vi "ClickConfocalSpot.vi"() -> ()   [LabVIEW 2013]
uses:
  <vilib>/Platform/TimedLoop/XDataNode/wakeup.ctl
  <vilib>/Platform/TimedLoop/XDataNode/XDNodeRunTimeDep.lvlib
  <vilib>/Platform/TimedLoop/XDataNode/nitl_modes.ctl
  <vilib>/Platform/TimedLoop/XDataNode/timing_clust.ctl
  <vilib>/Platform/TimedLoop/XDataNode/XDataNode.xnode
  <vilib>/Utility/miscctls.llb/LVPoint32TypeDef.ctl
  <vilib>/Utility/miscctls.llb/LVMinMaxIncTypeDef.ctl
panel:
  in  "BD 2 Frequency 2 (MHz)":dbl=26.0 min=60.0 max=90.0 step=1.0 format="%#_6p"
  in  "BD 1 Frequency 2 (MHz)":dbl=90.0 caption="T2 X (MHz)" min=60.0 max=90.0 step=1.0 format="%#_6p"
  in  "BD 2 Frequency 3 (MHz)":dbl=26.0 min=60.0 max=90.0 step=1.0 format="%#_6p"
  in  "BD 1 Frequency 3 (MHz)":dbl=70.0 min=60.0 max=90.0 step=1.0 format="%#_6p"
  in  "Trap Delta (MHz)":dbl=20.0 step=1.0
  out "X RF Frequency Limits (MHz)":T1={"Minimum"=60.0, "Maximum"=90.0, "Increment"=1.0}
  out "Y RF Frequency Limits (MHz)":T1={"Minimum"=60.0, "Maximum"=90.0, "Increment"=1.0}
  out "Manipulating Trap":bool
  in  "BD 1 Frequency 1 (MHz)":dbl=70.0 caption="T1 X (MHz)" min=60.0 max=90.0 step=1.0 format="%#_6p"
  in  "BD 2 Frequency 1 (MHz)":dbl=26.0 min=60.0 max=90.0 step=1.0 format="%#_6p"
  out "Initial Y":dbl=2.5691326639606933
  out "Initial X":dbl=1.6310662274449115
  in  "Scan steps (MCL)":u64=40 caption="Scan steps (x)"
  in  "Scan lines (y)":u64=20
  out "Actual MCL Inc (V)":dbl=0.14099551377910702
  out "Coords":T2
  in  "Manipulation Scaling":cluster{"Horizontal":dbl, "Vertical":dbl}={"Horizontal"=0.075, "Vertical"=0.01}
  in  "Manip. X?":bool=TRUE
  in  "Manip. Y?":bool
  in  "Limit Max (MHz)":dbl=16.0 caption="Max (MHz)"
  in  "Limit Min (MHz)":dbl=10.0 caption="Min (MHz)"
  in  "Limits Enable":bool=TRUE caption="Enable"
  in  "Force Manip Abort":bool
  out "Pointer X (V)":dbl=4.635613485356835 format="%_3g"
  out "Pointer Y (V)":dbl=4.0025870540482815 format="%_3g"
  in  "Set Confocal Spot (X-Y)":bool
  in  "Set Y Only":bool
  in  "Set X Only":bool
  in  "Scripts":T3(tab)=enum."Calibration"
  in  "Negate trap 2 force":bool
  in  "Take full offset\n data for display":bool=TRUE
  in  "Pause at Closest Delta (s)":dbl
  in  "Move to Delta 2 (MHz)":dbl=41.0
  in  "Attempt Limit":dbl=30.0 caption="Limit"
  out "Attempts":dbl=1.0
  in  "Wait Before Save (s)":u32=1
  in  "Fish for Tether":bool
  in  "Closest Delta (MHz)":dbl=13.0 step=0.25
  in  "Stop F (pN)":dbl=10.0
  in  "Then...":string(combo)="2"
  in  "Move to Delta 1 (MHz)":dbl=15.0
  in  "Tether Alarm?":bool=TRUE
  in  "TA Cancel Save?":bool=TRUE
  in  "TA Green Off?":bool=TRUE
  in  "Raster Set Upon Tether":u32=1
  in  "Save at end (5, 6)":bool
  in  "APD to Watch":bool
  out "Duration (s)":dbl
  in  "Action":string(combo)="Yank"
  in  "Fl. Delta Thresh. (kHz)":dbl=0.6
  out "Waiting":bool
  out "Fl. High":bool
  in  "N pts to average":u16=6
  in  "Yank Delay (s)":dbl=3.5
  in  "Yank to Delta Array (MHz)":dbl[](array[numeric])=[16.3, 15.85, 14.85]
  in  "N Array El":u8=3 min=1 step=1
  in  "Random Choice":bool=TRUE
  in  "Force Yank":bool
  in  "Force Reset":bool
  in  "Profile":bool
  # "After"
  # "During"
  # "Trap On?"
  # "BD Flow ON?"
  # "Samp Flow ON?"
  # "1"
  # "2"
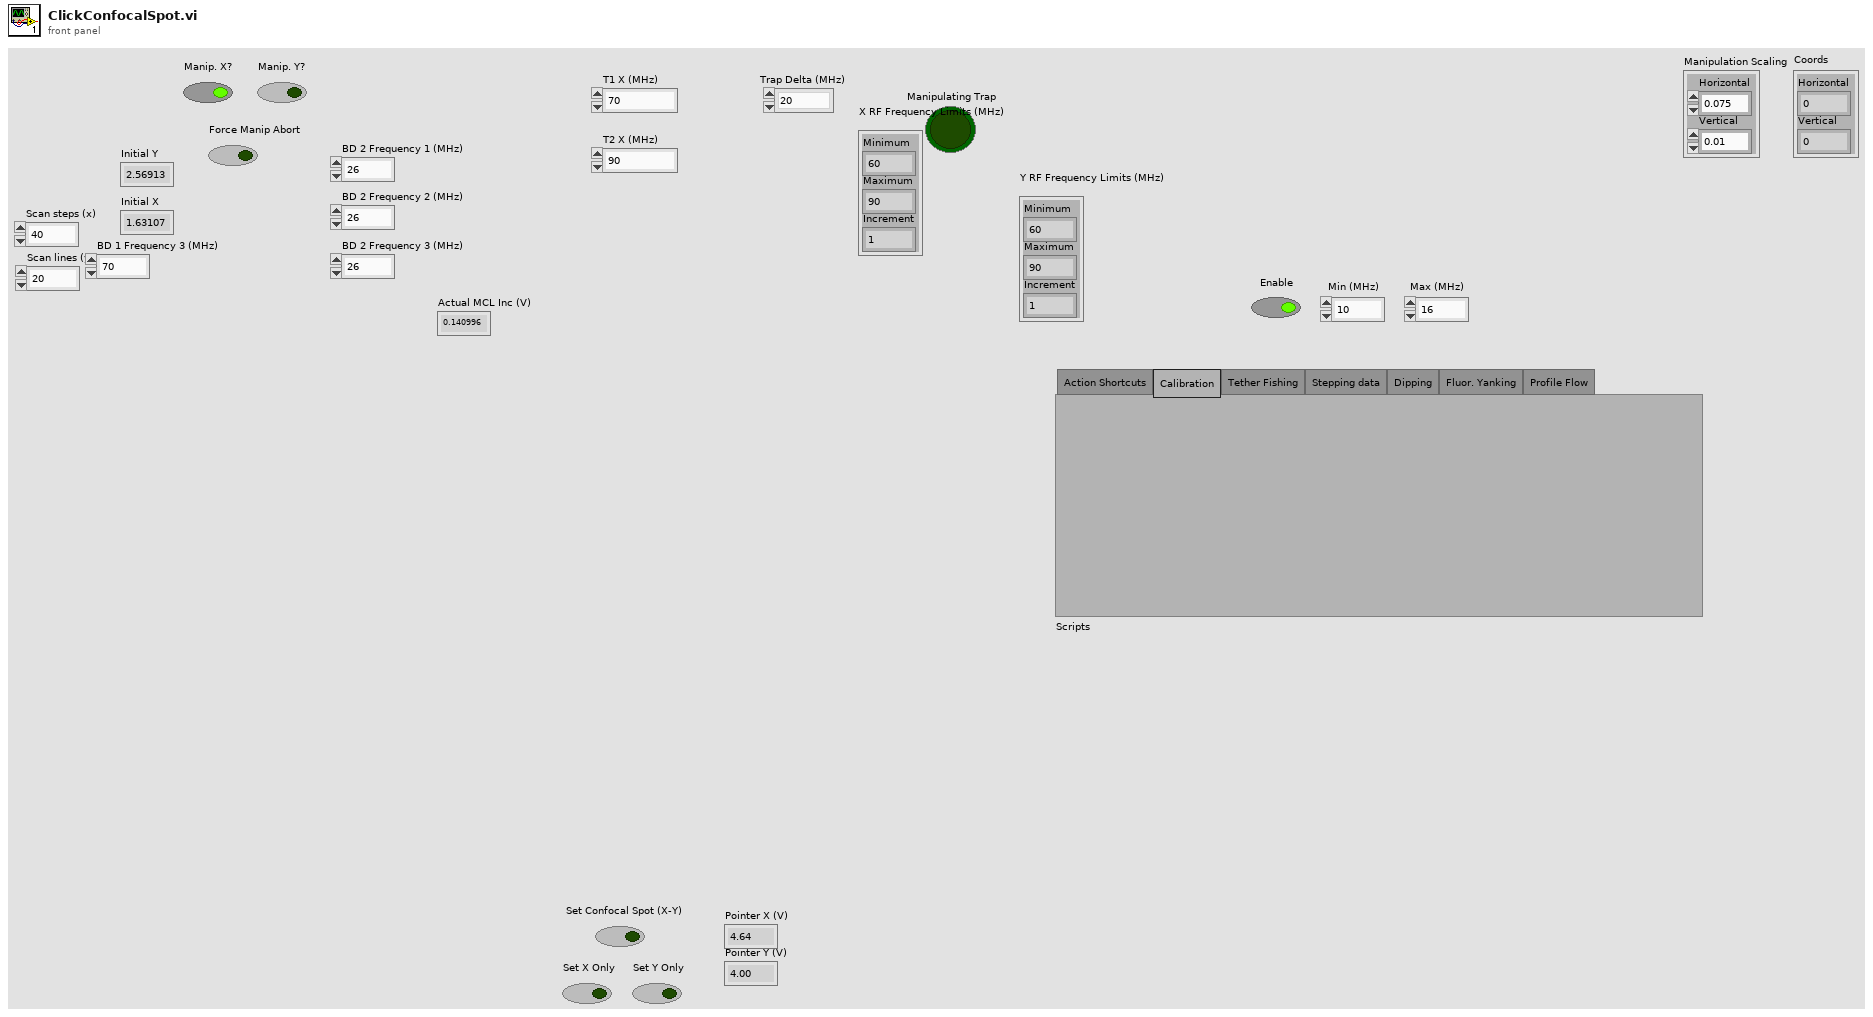
[diagram p1: front panel]
types:
  T1 = typedef "LVMinMaxIncTypeDef.ctl" = cluster{"Minimum":dbl, "Maximum":dbl, "Increment":dbl}
  T2 = typedef "LVPoint32TypeDef.ctl" = cluster{"Horizontal":i32, "Vertical":i32}
  T3 = enum32{"Action Shortcuts", "Calibration", "Tether Fishing", "Stepping data", "Dipping", "Fluor. Yanking", "Profile Flow"}
  T4 = typedef "XDNodeRunTimeDep.lvlib/timing_clust.ctl" = cluster{"Expected End [f-1]":u64, "Actual End [f-1]":u64, "Finished Late? [f-1]":bool, "Expected End [i-1]":u64, "Actual End [i-1]":u64, "Finished Late? [i-1]":bool, "Expected Start [i]":u64, "Actual Start [i]":u64, "Expected Start [f]":u64, "Actual Start [f]":u64, "Source Name":string, "Structure Name":string, "Period":i64, "Deadline":i64, "Offset":i64, "Start":i64, "Priority":i32, "Timeout":i32, "Mode":T5, "Wakeup Reason":T6, "Error":errorcluster, "Source Type":string, "Secondary Source Type":string, "Global End Time":u64, "Global Start Time":u64, "Frame Duration":u64, "Iteration Duration":u64, "Assigned CPU":i32, "I/O Scan Engine Mode":u32}
  T5 = typedef "XDNodeRunTimeDep.lvlib/nitl_modes.ctl" = enum32{"No Change", "Process missed periods, maintain original phase", "Discard missed periods, maintain original phase", "Process missed periods, ignore original phase", "Discard missed periods, ignore original phase"}
  T6 = typedef "XDNodeRunTimeDep.lvlib/wakeup.ctl" = enum32{"Normal", "Aborted", "Asynchronous wakeup", "Timing source error", "Timed loop error", "Timeout"}
  T7 = cluster{"Left":i32, "Top":i32, "Width":u32, "Height":u32}
  T8 = cluster{cluster{"Left":i32, "Top":i32, "Width":u32, "Height":u32}}[]
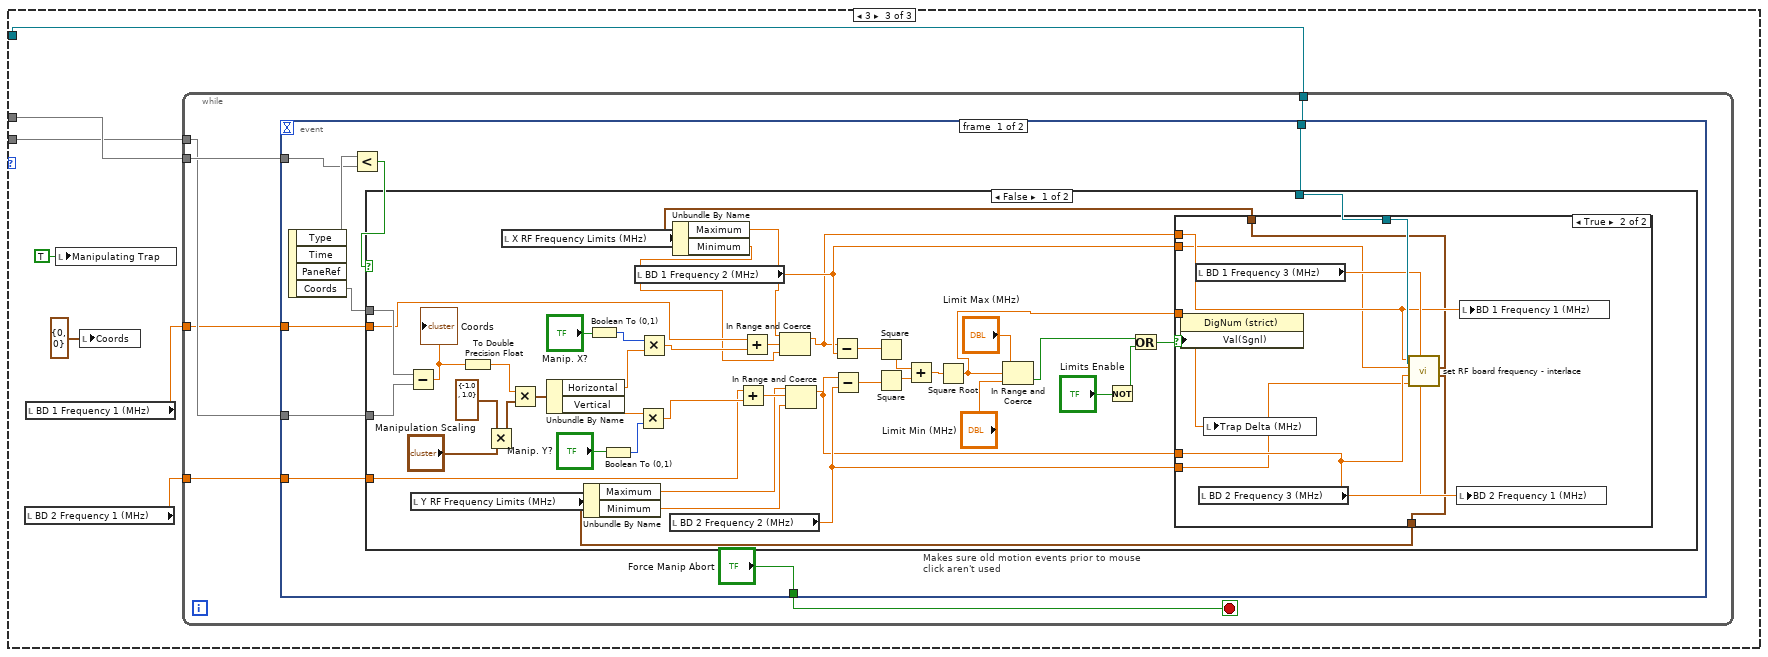
[diagram p7: hidden frame]
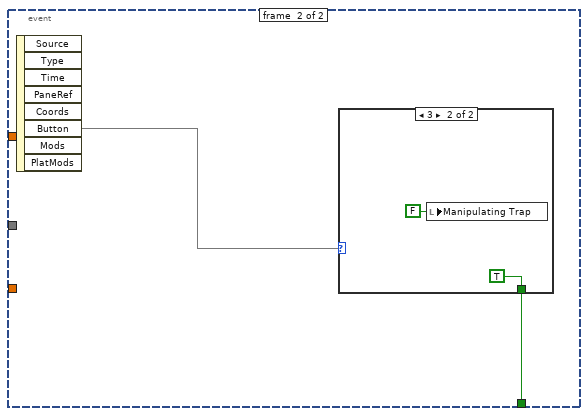
[diagram p10: hidden frame]
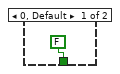
[diagram p11: hidden frame]
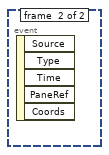
[diagram p12: hidden frame]
diagram:
  n1 = node-c288() -> (w2:T4)  [unwired: 4 out]
  n2 = timed-loop "Mouse control: trap position (AOM deflection), set confocal spot from image" {
    tunnel: [w4] -> _
    tunnel: _ -> [w3]
    timing: w2 -> [_]
    timing-out: [_] -> w1
    stop <- w4 stop-if-true
    n3 = node-c288() -> ()  [unwired: 2 out]
    n4 = event shown="[0]" {
      selector: _ -> [_ _]
      dyn-events: _ -> [_ _]
      timeout: _ -> [_ _]
      tunnel: w3 -> [w7 _]
      event #0 {
        n5 = event-data() -> ("Time"=w9, "Coords"=w8, "Button"=w10)  [unwired: 6 out]
        n6 = case shown="1" w10 {
          tunnel: w9 -> [_ _ w113]
          tunnel: w8 -> [_ w47 w111]
          tunnel: w7 -> [_ _ w109]
          frame 0, Default {
          }
          frame 1 {
            n7 = property on="Property Node" class="ImageControl"() -> ("Displayed Image Position"=w17:cluster{"Left":i32, "Top":i32})  [unwired: 2 in, 2 out]
            n8 = property on="Property Node" class="ImageControl"() -> ("Displayed Image Position"=w46:cluster{"Left":i32, "Top":i32})  [unwired: 2 in, 2 out]
            n9 = property on="Property Node" class="ImageControl"() -> ("Displayed Image Position"=w43:cluster{"Left":i32, "Top":i32})  [unwired: 2 in, 2 out]
            n10 = property on="Property Node" class="ImageControl"() -> ("Displayed Image Position"=w42:cluster{"Left":i32, "Top":i32})  [unwired: 2 in, 2 out]
            n11 = property on="Property Node" class="ImageControl"() -> ("Displayed Image Size"=w16:cluster{"Width":u32, "Height":u32})  [unwired: 2 in, 2 out]
            n12 = property on="Property Node" class="ImageControl"() -> ("Displayed Image Size"=w44:cluster{"Width":u32, "Height":u32})  [unwired: 2 in, 2 out]
            n13 = property on="Property Node" class="ImageControl"() -> ("Displayed Image Size"=w45:cluster{"Width":u32, "Height":u32})  [unwired: 2 in, 2 out]
            n14 = property on="Property Node" class="ImageControl"() -> ("Displayed Image Size"=w41:cluster{"Width":u32, "Height":u32})  [unwired: 2 in, 2 out]
            n15 = Unbundle By Name(w16) -> ("Width"=w13:u32, "Height"=w12:u32)
            n16 = Unbundle By Name(w17) -> ("Left"=w15:i32, "Top"=w14:i32)
            n17 = Unbundle By Name(w44) -> ("Width"=w38:u32, "Height"=w37:u32)
            n18 = Unbundle By Name(w45) -> ("Width"=w34:u32, "Height"=w33:u32)
            n19 = Unbundle By Name(w41) -> ("Width"=w30:u32, "Height"=w29:u32)
            n20 = Unbundle By Name(w46) -> ("Left"=w40:i32, "Top"=w39:i32)
            n21 = Unbundle By Name(w43) -> ("Left"=w36:i32, "Top"=w35:i32)
            n22 = Unbundle By Name(w42) -> ("Left"=w32:i32, "Top"=w31:i32)
            n23 = Bundle("Left"=w15, "Top"=w14, "Width"=w13, "Height"=w12) -> (w11:T7)  [unwired: 1 in]
            n24 = Bundle("Left"=w40, "Top"=w39, "Width"=w38, "Height"=w37) -> (w28:T7)  [unwired: 1 in]
            n25 = Bundle("Left"=w36, "Top"=w35, "Width"=w34, "Height"=w33) -> (w27:T7)  [unwired: 1 in]
            n26 = Bundle("Left"=w32, "Top"=w31, "Width"=w30, "Height"=w29) -> (w26:T7)  [unwired: 1 in]
            n27 = Build Cluster Array(w11, w28, w27, w26) -> (w25:T8)
            n28 = for {
              tunnel: w47 -> [w58]
              tunnel: w25 -> [w59] mode=indexing
              shift-right: [w56] -> w23
              shift-left: TRUE -> [w57]
              shift-right: [w55] -> w21
              shift-left: _ -> [w51]
              shift-right: [w54] -> w20
              shift-left: _ -> [w50]
              shift-right: [w53] -> w19
              shift-left: _ -> [w49]
              shift-right: [w52] -> w18
              shift-left: _ -> [w48]
              n29 = case shown="True" w57 {
                selector: w57 -> [w64 _]
                tunnel: w59 -> [_ w73]
                tunnel: w58 -> [_ w71]
                tunnel: [w64 w69] -> w56
                tunnel: [w63 w68] -> w55
                tunnel: [w62 w67] -> w54
                tunnel: [w61 w66] -> w53
                tunnel: [w60 w65] -> w52
                tunnel: w51 -> [w63 _]
                tunnel: w50 -> [w62 _]
                tunnel: w49 -> [w61 _]
                tunnel: w48 -> [w60 _]
                frame False {
                }
                frame True {
                  n30 = Unbundle(w73) -> (w72:T7)
                  n31 = call "isclickinwindow.vi"("Image Param"=w72, "Point32"=w71) -> ("4 Y"=w65:i32, "3 Height"=w66:i32, "2 X"=w67:i32, "1 Width"=w68:i32, "In image?"=w70:bool)  [unwired: 1 in]
                  n32 = Not(x=w70) -> (.not. x?=w69:bool)
                }
              }
            }
            n33 = Not(x=w23) -> (.not. x?=w22:bool)
            n34 = case shown="True" w22 {
              tunnel: w20 -> [_ w86]
              tunnel: w18 -> [_ w85]
              tunnel: w21 -> [_ w84]
              tunnel: w19 -> [_ w83]
              frame False {
              }
              frame True {
                w79 = FALSE ("Get Point")
                n35 = local read "Scan lines (y)"() -> (w88:u64)
                n36 = local read "Actual MCL Inc (V)"() -> (w80:dbl)
                n37 = local read "Scan steps (MCL)"() -> (w87:u64)
                n38 = Divide "Y Pix/step"(x=w83, y=w88) -> (x/y=w95:dbl)
                n39 = Divide "Y V/pix"(x=w80, y=w95) -> (x/y=w94:dbl)
                n40 = Divide "Y half step offset"(x=w80, y=2.0) -> (x/y=w96:dbl)
                n41 = Divide "X pix/step"(x=w84, y=w87) -> (x/y=w93:dbl)
                n42 = Negate(x=w96) -> (-x=w97:dbl)
                n43 = local read "Initial Y"() -> (w103:dbl)
                n44 = Multiply(x=w85, y=w94) -> (x*y=w104:dbl)
                n45 = Divide "X half step offset"(x=w80, y=2.0) -> (x/y=w90:dbl)
                n46 = Divide "X V/pix"(x=w80, y=w93) -> (x/y=w92:dbl)
                n47 = Multiply(x=w80, y=w87) -> (x*y=w99:dbl)
                n48 = Compound Arithmetic op=ADD(w97, w104, w103) -> (w81:dbl)
                "Pointer Y (V)" <- w81
                n49 = Multiply(x=w92, y=w86) -> (x*y=w101:dbl)
                n50 = Negate(x=w90) -> (-x=w89:dbl)
                n51 = local read "Initial X"() -> (w102:dbl)
                n52 = Negate(x=w101) -> (-x=w100:dbl)
                n53 = Compound Arithmetic op=ADD(w89, w99, w102, w100) -> (w82:dbl)
                "Pointer X (V)" <- w82
                n54 = Or(x="Set X Only", y="Set Confocal Spot (X-Y)") -> (x .or. y?=w75:bool)
                n55 = Or(x="Set Confocal Spot (X-Y)", y="Set Y Only") -> (x .or. y?=w74:bool)
                n56 = case shown="True" w75 {
                  tunnel: w82 -> [_ w105]
                  frame False {
                  }
                  frame True {
                    n57 = property on="Property Node" class="Slide (strict)"("Val(Sgnl)"=w105) -> ()  [unwired: 2 in, 2 out]
                  }
                }
                n58 = case shown="True" w74 {
                  tunnel: w81 -> [_ w106]
                  frame False {
                  }
                  frame True {
                    n59 = property on="Property Node" class="Slide (strict)"("Val(Sgnl)"=w106) -> ()  [unwired: 2 in, 2 out]
                  }
                }
                n60 = local write "Set Confocal Spot (X-Y)"(w79) -> ()
                n61 = local write "Set X Only"(w79) -> ()
                n62 = local write "Set Y Only"(w79) -> ()
              }
            }
          }
          frame 3 {
            n63 = local read "BD 2 Frequency 1 (MHz)"() -> (w107:dbl)
            n64 = local read "BD 1 Frequency 1 (MHz)"() -> (w108:dbl)
            n65 = local write "Manipulating Trap"(TRUE ("Manipulating Trap")) -> ()
            n66 = local write "Coords"(T2 {"Horizontal"=0, "Vertical"=0} ("Coords")) -> ()
            n67 = while {
              tunnel: w113 -> [w118]
              tunnel: w111 -> [w117]
              tunnel: w109 -> [w116]
              tunnel: w108 -> [w115]
              tunnel: w107 -> [w114]
              stop <- w119 stop-if-true
              n68 = event shown="[0]" {
                selector: _ -> [_ _]
                dyn-events: _ -> [_ _]
                timeout: _ -> [_ _]
                tunnel: ["Force Manip Abort" w183] -> w119
                tunnel: w118 -> [w126 _]
                tunnel: w117 -> [w124 _]
                tunnel: w116 -> [w123 _]
                tunnel: w115 -> [w122 _]
                tunnel: w114 -> [w121 _]
                event #0 {
                  n69 = event-data() -> ("Time"=w127, "Coords"=w128)  [unwired: 3 out]
                  n70 = Less?(x=w127, y=w126) -> (x < y?=w125:bool)
                  n71 = case "Makes sure old motion events prior to mouse click aren't used" shown="False" w125 {
                    tunnel: w128 -> [w170 _]
                    tunnel: w124 -> [w171 _]
                    tunnel: w123 -> [w148 _]
                    tunnel: w122 -> [w144 _]
                    tunnel: w121 -> [w143 _]
                    frame False {
                      n72 = Subtract(x=w170, y=w171) -> (x-y=w169:dbl)
                      "Coords" <- w169
                      n73 = local read "Y RF Frequency Limits (MHz)"() -> (w129:T1)
                      n74 = To Double Precision Float(number=w169) -> (double precision float=w168:dbl)
                      n75 = Multiply(x=cluster{"Horizontal":dbl, "Vertical":dbl} {"Horizontal"=-1.0, "Vertical"=1.0}, y="Manipulation Scaling") -> (x*y=w164:cluster{"Horizontal":dbl, "Vertical":dbl})
                      n76 = local read "X RF Frequency Limits (MHz)"() -> (w130:T1)
                      n77 = Multiply(x=w168, y=w164) -> (x*y=w166:cluster{"Horizontal":dbl, "Vertical":dbl})
                      n78 = Unbundle By Name(w166) -> ("Horizontal"=w161:dbl, "Vertical"=w165:dbl)
                      n79 = Unbundle By Name(w129) -> ("Maximum"=w132:dbl, "Minimum"=w131:dbl)
                      n80 = Boolean To (0,1)(Boolean="Manip. X?") -> (0, 1=w159:i16)
                      n81 = Boolean To (0,1)(Boolean="Manip. Y?") -> (0, 1=w156:i16)
                      n82 = local read "BD 1 Frequency 2 (MHz)"() -> (w146:dbl)
                      n83 = Multiply(x=w165, y=w156) -> (x*y=w158:dbl)
                      n84 = Multiply(x=w159, y=w161) -> (x*y=w162:dbl)
                      n85 = local read "BD 2 Frequency 2 (MHz)"() -> (w145:dbl)
                      n86 = Unbundle By Name(w130) -> ("Maximum"=w134:dbl, "Minimum"=w133:dbl)
                      n87 = Add(x=w143, y=w158) -> (x+y=w136:dbl)
                      n88 = Add(x=w144, y=w162) -> (x+y=w138:dbl)
                      n89 = In Range and Coerce(upper limit=w134, x=w138, lower limit=w133) -> (coerced(x)=w137:dbl)  [unwired: 1 out]
                      n90 = In Range and Coerce(upper limit=w132, x=w136, lower limit=w131) -> (coerced(x)=w135:dbl)  [unwired: 1 out]
                      n91 = Subtract(x=w137, y=w146) -> (x-y=w155:dbl)
                      n92 = Subtract(x=w135, y=w145) -> (x-y=w154:dbl)
                      n93 = Square(x=w155) -> (x^2=w153:dbl)
                      n94 = Square(x=w154) -> (x^2=w152:dbl)
                      n95 = Add(x=w153, y=w152) -> (x+y=w151:dbl)
                      n96 = Square Root(x=w151) -> (sqrt(x)=w147:dbl)
                      n97 = In Range and Coerce(upper limit="Limit Max (MHz)", x=w147, lower limit="Limit Min (MHz)") -> (In Range?=w140:bool)  [unwired: 1 out]
                      n98 = Not(x="Limits Enable") -> (.not. x?=w139:bool)
                      n99 = Or(x=w140, y=w139) -> (x .or. y?=w141:bool)
                      n100 = case shown="True" w141 {
                        tunnel: w148 -> [_ w181]
                        tunnel: w147 -> [_ w172]
                        tunnel: w137 -> [_ w179]
                        tunnel: w146 -> [_ w178]
                        tunnel: w135 -> [_ w177]
                        tunnel: w145 -> [_ w176]
                        tunnel: w130 -> [_ w174]
                        tunnel: w129 -> [_ w173]
                        frame False {
                        }
                        frame True {
                          n101 = property on="Property Node" class="DigNum (strict)"("Val(Sgnl)"=w172) -> ()  [unwired: 2 in, 2 out]
                          n102 = local read "BD 1 Frequency 3 (MHz)"() -> (w180:dbl)
                          n103 = local read "BD 2 Frequency 3 (MHz)"() -> (w175:dbl)
                          n104 = local write "Trap Delta (MHz)"(w172) -> ()
                          n105 = call "set RF board frequency - interlace.vi"("Board 2 Frequency Limits"=w173, "Board 1 Frequency Limits"=w174, "FPGA VI Reference In"=w181, "Board 2 Frequency 3 (MHz)"=w175, "Board 1 Frequency 3 (MHz)"=w180, "Board 2 Frequency 2 (MHz)"=w176, "Board 2 Frequency 1 (MHz)"=w177, "Board 1 Frequency 2 (MHz)"=w178, "Board 1 Frequency 1  (MHz)"=w179) -> ()  [unwired: 1 in, 2 out]
                          n106 = local write "BD 2 Frequency 1 (MHz)"(w177) -> ()
                          n107 = local write "BD 1 Frequency 1 (MHz)"(w179) -> ()
                        }
                      }
                    }
                    frame True {
                    }
                  }
                }
                event #1 {
                  n108 = event-data() -> ("Button"=w182)  [unwired: 8 out]
                  n109 = case shown="3" w182 {
                    tunnel: [FALSE TRUE] -> w183
                    frame 0, Default {
                    }
                    frame 3 {
                      n110 = local write "Manipulating Trap"(FALSE ("Manipulating Trap")) -> ()
                    }
                  }
                }
              }
            }
          }
        }
      }
      event #1 {
        n111 = event-data() -> ()  [unwired: 6 out]
      }
    }
    n112 = local read item#-1() -> (w4)
    n113 = node-c288() -> ()  [unwired: 2 out]
  }
  n114 = node-c288(w1) -> ()  [unwired: 1 out]
